vi "integral plot.vi"(8 "error in (no error)":errorcluster, 10 "Array path":path[](array[path]), 11 "Data channel":u16) -> (0 "error out":errorcluster, 3 "Array":cluster{"Data out":dbl[], "Data out":dbl[]}[](array[cluster]))   [LabVIEW 2023]
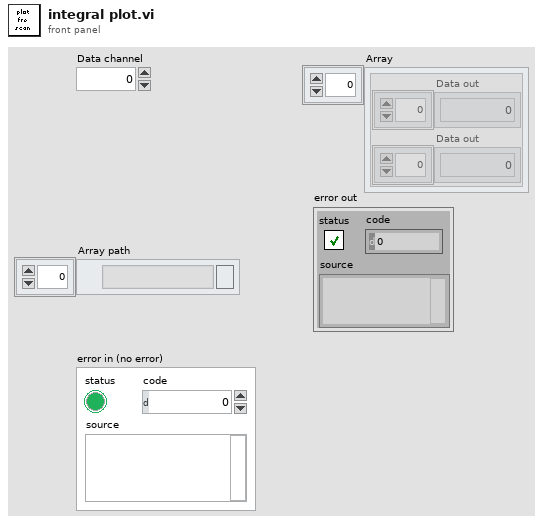
[diagram p1: front panel]
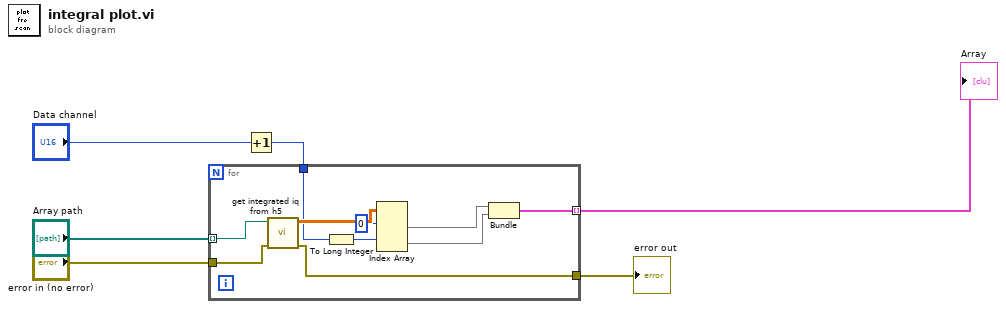
[diagram p0: block diagram]
diagram:
  n1 = Increment(x="Data channel") -> (x+1=w4:u16)
  n2 = for {
    tunnel: "error in (no error)" -> [w16]
    tunnel: w4 -> [w12]
    tunnel: [w9] -> w5 mode=indexing
    tunnel: "Array path" -> [w8] mode=indexing
    tunnel: [w7] -> w1
    n3 = call "get integrated iq from h5.vi"("error in (no error)"=w16, "path"=w8) -> ("error out"=w7:errorcluster, "Data out"=w15:dbl[][])  [unwired: 8 in]
    n4 = To Long Integer(number=w12) -> (32bit integer=w11:i32)
    n5 = Index Array(array=w15, index (row) #1=0 ("index (row)"), index (row) #2=w11) -> (element #1=w13:dbl[], element #2=w10:dbl[])  [unwired: 2 in]
    n6 = Bundle("Data out"=w13, "Data out"=w10) -> (w9:cluster{"Data out":dbl[], "Data out":dbl[]})  [unwired: 1 in]
  }
  "Array" <- w5
  "error out" <- w1
